vi "Initialize Motor Communication Val.vi"(8 "error in (no error)":errorcluster) -> (0 "error out":errorcluster, 3 "motor communication val out":refnum<class "NI_Robotics_Motor Communication Val.lvclass">)   [LabVIEW 2017, in "NI_Robotics_Motor Communication Val.lvclass"]
uses:
  <vilib>/robotics/Actuation/Motor Communication Val/NI_Robotics_Motor Communication Val.lvclass
  c:/Program Files (x86)/National Instruments/LabVIEW 2017/vi.lib/robotics/Actuation/Motor Communication/NI_Robotics_Motor Communication.lvclass
  <vilib>/robotics/Actuation/Motor Communication/Motor State Value.ctl
  <vilib>/robotics/Actuation/Motor Communication/Motor State Mode.ctl
  <vilib>/robotics/Actuation/Motor Communication Val/NI_Robotics_Motor Communication Val.lvclass/NI_Robotics_Motor Communication Val.ctl
  <vilib>/robotics/Actuation/Motor Communication/NI_Robotics_Motor Communication.lvclass/NI_Robotics_Motor Communication.ctl
  <vilib>/robotics/Actuation/Motor Communication/NI_Robotics_Motor Communication.lvclass
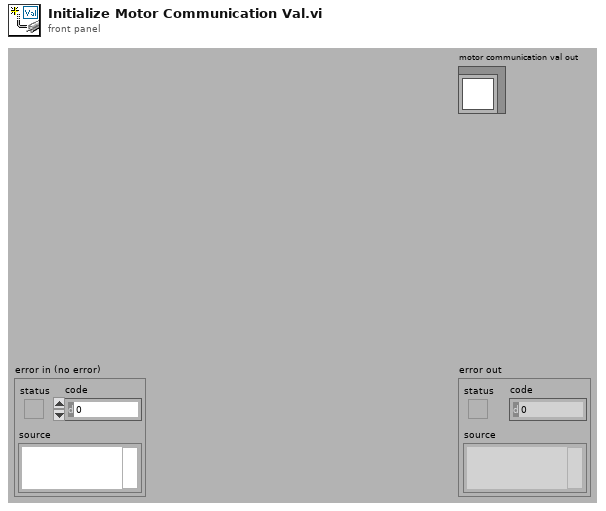
[diagram p1: front panel]
types:
  T1 = typedef "NI_Robotics_Motor Communication.lvclass/Motor State Value.ctl" = cluster{"angle":dbl, "velocity":dbl, "state mode":T2}
  T2 = typedef "NI_Robotics_Motor Communication.lvclass/Motor State Mode.ctl" = u16
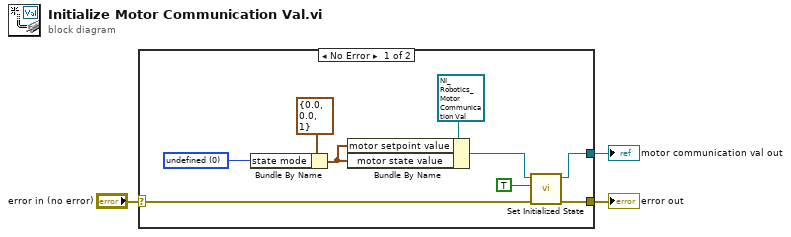
[diagram p0: block diagram]
diagram:
  n1 = case shown="No Error" "error in (no error)" {
    selector: "error in (no error)" -> [w8 w13]
    tunnel: [w7 w13] -> w2
    tunnel: [w4 _] -> w1
    frame No Error {
      w10 = T2 0 items=["undefined", "angle", "velocity"] ("state mode")
      n2 = Bundle By Name(cluster=T1 {"angle"=0.0, "velocity"=0.0, "state mode"=1} ("state value"), "state mode"=w10) -> (w9:T1)
      n3 = Bundle By Name(cluster=refnum<class "NI_Robotics_Motor Communication Val.lvclass"> refnum ("NI_Robotics_Motor Communication Val in"), "motor setpoint value"=w9, "motor state value"=w9) -> (w5:refnum<class "NI_Robotics_Motor Communication Val.lvclass">)
      n4 = call <vilib>:"Set Initialized State.vi"("error in (no error)"=w8, "initialized"=TRUE, "motor communication in"=w5) -> ("error out"=w7:errorcluster, "motor communication out"=w4:refnum<class "NI_Robotics_Motor Communication Val.lvclass">)  [unwired: 7 in]
    }
    frame Error {
    }
  }
  "error out" <- w2
  "motor communication val out" <- w1
